vi "Auc.vi"(8 "error in (no error)":errorcluster caption="entrée d'erreur (pas d'erreur)", 10 "y":string[][](array[string]), 11 "x":string[][](array[string])) -> (0 "error out":errorcluster caption="sortie d'erreur", 3 "Score":string)   [LabVIEW 2020]
doc: "Compute Area Under the Curve (AUC) using the trapezoidal rule\n\nThis is a general function, given points on a curve. For computing the area under the ROC-curve, see roc_auc_score. For an alternative way to summarize a precision-recall curve, see average_precision_score.\n\n\nParameters :\n\n- x : array, shape = [n]\nx coordinates. These must be either monotonic increasing or monotonic decreasing.\n\n- y : array, shape = [n]\ny coordinates.\n\nReturns : \n\n- auc : float"
uses:
  Auc.lvclass
panel:
  out "Auc.lvclass":refnum<class "Auc.lvclass">
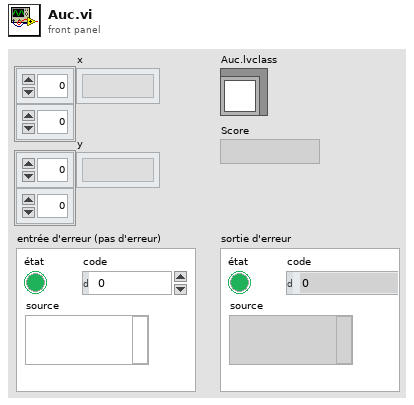
[diagram p1: front panel]
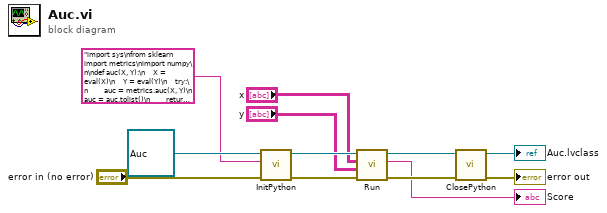
[diagram p0: block diagram]
diagram:
  n1 = call-dynamic "InitPython.vi"("error in (no error)"="error in (no error)", "Python Instruction"="import sys\nfrom sklearn import metrics\nimport numpy\n\ndef auc(X, Y):\n    X = eval(X)\n    Y = eval(Y)\n    try:\n        auc = metrics.auc(X, Y)\n        auc = auc.tolist()\n        return str(auc)\n    except:\n        erreur = sys.exc_info()\n        typerr = u\"%s\" % (erreur[0])\n        typerr = typerr[typerr.find(\"'\")+1:typerr.rfind(\"'\")]\n        msgerr = u\"%s\" % (erreur[1])\n        message = str('/!\\\\ {0} : {1}'. format(typerr,msgerr))\n        return message", "Scikit-learn en entrée"=refnum<class "Auc.lvclass"> refnum ("Auc.lvclass")) -> ("error out"=w8:errorcluster, "Scikit-learn en sortie"=w9:refnum<class "Auc.lvclass">)  [unwired: 7 in]
  n2 = call-dynamic "Run.vi"("error in (no error)"=w8, "y"="y", "x"="x", "Auc.lvclass"=w9) -> ("error out"=w6:errorcluster, "Score"=→"Score":string, "Auc.lvclass"=w7:refnum<class "Auc.lvclass">)  [unwired: 5 in]
  n3 = call-dynamic "ClosePython.vi"("error in (no error)"=w6, "Scikit-learn en entrée"=w7) -> ("error out"=→"error out":errorcluster, "Scikit-learn en sortie"=→"Auc.lvclass":refnum<class "Auc.lvclass">)  [unwired: 8 in]
